vi "HFRR ADV v05.vi"() -> ()   [LabVIEW 2025] (continued)
            n2732 = Path To String(path=w3785) -> (string=w3768:string)
            n2733 = while {
              tunnel: w3777 -> [w3789]
              i -> [w3786]
              stop <- w3787 continue-if-true
              (unwired) TRUE ("line mode (F)")
              n2734 = Read from Text File "Read File"(file (use dialog)=w3789) -> (text=w3788:string)  [unwired: 3 in, 3 out]
              n2735 = local write "Numeric 16"(w3786) -> ()
              n2736 = String Length(string=w3788) -> (length=w3791:i32)
              n2737 = Greater?(x=w3791, y=1) -> (0:w3787:bool)
            }
            n2738 = local write "String 29"(w3768) -> ()
            n2739 = Search and Replace String(input string=w3768, search string=".duf", replace string=".dgf" ("replace string (\"\")")) -> (result string=→"String Indicator 4":string)  [unwired: 5 in, 3 out]
            n2740 = Match Pattern(string=w3783, regular expression=".dwm") -> (before substring=w3767:string)  [unwired: 1 in, 3 out]
            "String Indicator" <- w3767
            n2741 = Match Pattern(string=w3768, regular expression=".dwm" ("substring (\"\")")) -> (before substring=w3769:string)  [unwired: 1 in, 3 out]
            "String Indicator 3" <- w3769
            n2742 = local write "TITTLE 2"(w3767) -> ()
            n2743 = String To Path(string=w3769) -> (path=w3776:path)
            "path" <- w3776
            n2744 = call <vilib>:"Read Characters From File.vi"("file path (dialog if empty)"=w3776, "start of read offset (chars.:0)"=60 ("start of read offset (chars.: 0)")) -> ("character string"=→"String Indicator 2":string)  [unwired: 4 in, 3 out]
          }
        }
        n2745 = call <vilib>:"Query Available Printers.vi"() -> ("system configured printers"=w3468:string[])  [unwired: 9 in, 2 out]
        "System Configured Printers 2" <- w3468
        n2746 = local read "OK Button 16"() -> (w3465:bool)
        n2747 = case shown="True" "OK Button 16" {
          frame False {
          }
          frame True {
            n2748 = stacked-sequence {
              frame #0 {
                n2749 = local read "Numeric 16"() -> (w3793:i32)
                n2750 = local write "Numeric 10"(w3793) -> ()
              }
              frame #1 {
                n2751 = local read "S.NO"() -> (→"s.NO":string)
                n2752 = local read "String 29"() -> (w3797:string)
                n2753 = String To Path(string=w3797) -> (path=w3796:path)
                n2754 = Open/Create/Replace File "Open File"(file path (use dialog)=w3796) -> (refnum out=w3798:refnum<file>)  [unwired: 5 in, 2 out]
                n2755 = for {
                  N: 16 -> [_]
                  tunnel: w3798 -> [w3805]
                  i -> [w3801]
                  (unwired) TRUE ("line mode (F)")
                  n2756 = Read from Text File "Read File"(file (use dialog)=w3805) -> (text=w3799:string)  [unwired: 3 in, 3 out]
                  n2757 = Match Pattern(string=w3799, regular expression="(") -> (after substring=w3804:string)  [unwired: 1 in, 3 out]
                  n2758 = Match Pattern(string=w3804, regular expression=")") -> (before substring=w3800:string)  [unwired: 1 in, 3 out]
                  n2759 = case shown="1" w3801 {
                    tunnel: w3800 -> [w3806 w3807 _ _ w3808 w3809 w3810 w3812 w3814 w3816 w3818 w3820 w3822 w3824 _]
                    tunnel: w3799 -> [_ _ _ _ _ _ _ _ _ _ _ _ _ _ _]
                    frame 0 {
                      "TITTLE" <- w3806
                    }
                    frame 1 {
                      "Sample ID" <- w3807
                    }
                    frame 2 {
                    }
                    frame 3 {
                    }
                    frame 4 {
                      "Test Date" <- w3808
                    }
                    frame 5 {
                      "Tested by" <- w3809
                    }
                    frame 6 {
                      n2760 = Fract/Exp String To Number(string=w3810) -> (number=→"Humidity before test 2":dbl)  [unwired: 3 in, 1 out]
                    }
                    frame 7 {
                      n2761 = Fract/Exp String To Number(string=w3812) -> (number=→"Temperature before test 2":dbl)  [unwired: 3 in, 1 out]
                    }
                    frame 8 {
                      n2762 = Fract/Exp String To Number(string=w3814) -> (number=→"Humidity after test 2":dbl)  [unwired: 3 in, 1 out]
                    }
                    frame 9 {
                      n2763 = Fract/Exp String To Number(string=w3816) -> (number=→"Temperature after test 2":dbl)  [unwired: 3 in, 1 out]
                    }
                    frame 10 {
                      n2764 = Fract/Exp String To Number(string=w3818) -> (number=→"MWSD 2":dbl)  [unwired: 3 in, 1 out]
                    }
                    frame 11 {
                      n2765 = Fract/Exp String To Number(string=w3820) -> (number=→"AVP 2":dbl)  [unwired: 3 in, 1 out]
                    }
                    frame 12 {
                      n2766 = Fract/Exp String To Number(string=w3822) -> (number=→"HCF 2":dbl)  [unwired: 3 in, 1 out]
                    }
                    frame 13 {
                      n2767 = Fract/Exp String To Number(string=w3824) -> (number=→"WS1.4 2":dbl)  [unwired: 3 in, 1 out]
                    }
                    frame 14, Default {
                    }
                  }
                }
              }
              frame #2 {
              }
            }
            n2768 = local write "OK Button 16"(FALSE ("OK Button 13")) -> ()
          }
        }
        n2769 = Index Array(array=w3468, index="Select Printer 3") -> (element=w3470:string)
        "Selected Printer" <- w3470
        n2770 = case shown="True" w3465 {
          frame False {
          }
          frame True {
            n2771 = flat-sequence {
              frame #0 {
              }
              frame #1 {
                n2772 = Wait (ms)(milliseconds to wait=u32 100) -> ()  [unwired: 1 out]
              }
              frame #2 {
                n2773 = local write "OK Button 16"(FALSE ("Print 3")) -> ()
              }
            }
          }
        }
        n2774 = case shown="True" "Print" {
          tunnel: w3470 -> [_ w3762]
          frame False {
          }
          frame True {
            (unwired) i16 6 ("width (-)")
            (unwired) "TESTED BY : "
            (unwired) "TESTED DATE :"
            (unwired) "SAMPLE ID : "
            (unwired) "SAMPLE DESIGN : "
            w3720 = "\r"
            w3737 = "\r"
            # "add image"
            n2775 = local read "Sample ID"() -> (w3710:string)
            n2776 = local read "Tested by"() -> (w3713:string)
            n2777 = local read "String 34"() -> (w3700:string)
            n2778 = local read "String 45"() -> (w3680:string)
            n2779 = local read "String 35"() -> (w3695:string)
            n2780 = local read "String 37"() -> (w3693:string)
            n2781 = local read "String 32"() -> (w3715:string)
            n2782 = local read "String 36"() -> (w3690:string)
            n2783 = local read "String 31"() -> (w3714:string)
            n2784 = local read "Test Date"() -> (w3711:string)
            n2785 = local read "String 33"() -> (w3716:string)
            n2786 = local read "String 38"() -> (w3686:string)
            n2787 = local read "String 39"() -> (w3683:string)
            n2788 = local write "Print"(FALSE ("Print FF")) -> ()
            n2789 = local read "S 39"() -> (w3698:string)
            n2790 = local read "S 38"() -> (w3705:string)
            n2791 = local read "Temperature before test 2"() -> (w3736:dbl)
            n2792 = local read "Temperature after test 2"() -> (w3726:dbl)
            n2793 = local read "Humidity before test 2"() -> (w3751:dbl)
            n2794 = local read "Humidity after test 2"() -> (w3735:dbl)
            n2795 = local read "MWSD 2"() -> (w3740:dbl)
            n2796 = local read "WS1.4 2"() -> (w3718:dbl)
            n2797 = Concatenate Strings("2)" ("string"), w3700) -> (w3701:string)
            n2798 = Concatenate Strings("3)" ("string"), w3698) -> (w3699:string)
            n2799 = Concatenate Strings("1)" ("string"), w3705) -> (w3704:string)
            n2800 = Concatenate Strings("4)" ("string"), w3695) -> (w3696:string)
            n2801 = Concatenate Strings("5)" ("string"), w3693) -> (w3692:string)
            n2802 = Concatenate Strings("6)" ("string"), w3690) -> (w3689:string)
            n2803 = Concatenate Strings("7)" ("string"), w3686) -> (w3687:string)
            n2804 = Concatenate Strings("8)" ("string"), w3683) -> (w3684:string)
            n2805 = local read "HCF 2"() -> (w3722:dbl)
            n2806 = local read "AVP 2"() -> (w3739:dbl)
            n2807 = local read "s.NO"() -> (w3681:string)
            n2808 = call <vilib>:"New Report.vi"("report type"=enum16{"Standard Report", "HTML"}."Standard Report") -> ("report out"=w3760:refnum<class "NI_report.lvclass">, "error out"=w3759:errorcluster)  [unwired: 13 in]
            n2809 = local read "TITTLE"() -> (w3712:string)
            n2810 = Concatenate Strings(w3737, w3680, w3681, w3737, w3715, w3710, w3737, w3714, w3711, w3737, w3716, w3713, w3737) -> (w3730:string)
            "test by" <- w3730
            n2811 = Number To Fractional String(number=w3736, width (-)=i16 6, precision (6)=i16 2) -> (F-format string=w3725:string)  [unwired: 1 in]
            n2812 = Number To Fractional String(number=w3735, width (-)=i16 6, precision (6)=i16 2) -> (F-format string=w3738:string)  [unwired: 1 in]
            n2813 = Number To Fractional String(number=w3751, width (-)=i16 6, precision (6)=i16 2) -> (F-format string=w3756:string)  [unwired: 1 in]
            n2814 = Number To Fractional String(number=w3740, width (-)=i16 6, precision (6)=i16 2) -> (F-format string=w3742:string)  [unwired: 1 in]
            n2815 = Number To Fractional String(number=w3726, width (-)=i16 6, precision (6)=i16 2) -> (F-format string=w3727:string)  [unwired: 1 in]
            n2816 = Number To Fractional String(number=w3739, width (-)=i16 6, precision (6)=i16 2) -> (F-format string=w3741:string)  [unwired: 1 in]
            n2817 = Number To Fractional String(number=w3722, width (-)=i16 6, precision (6)=i16 2) -> (F-format string=w3721:string)  [unwired: 1 in]
            n2818 = Number To Fractional String(number=w3718, precision (6)=i16 2) -> (F-format string=w3717:string)  [unwired: 2 in]
            n2819 = call-dynamic "Set Report Header Text.vi"("report in"=w3760, "center header text"=w3712, "error in (no error)"=w3759) -> ("report out"=w3731:refnum<class "NI_report.lvclass">, "error out"=w3732:errorcluster)  [unwired: 11 in]
            n2820 = Concatenate Strings(w3720, w3704, w3756, w3720, w3701, w3725, w3720, w3699, w3738, w3720, w3696, w3727, w3720, w3692, w3742, w3720, w3689, w3741, w3720, w3687, w3721, w3720, w3684, w3717) -> (w3708:string)
            "export 2" <- w3708
            n2821 = call-poly <vilib>:"Append Report Text.vi"("report in"=w3731, "text"=w3730, "error in (no error)"=w3732) -> ("report out"=w3734:refnum<class "NI_report.lvclass">, "error out"=w3733:errorcluster)  [unwired: 9 in, 2 out]
            n2822 = local read "test by"() -> (w3707:string)
            n2823 = local read "TITTLE"() -> (w3709:string)
            n2824 = call-poly <vilib>:"Append Report Text.vi"("report in"=w3734, "error in (no error)"=w3733) -> ("report out"=w3755:refnum<class "NI_report.lvclass">, "error out"=w3753:errorcluster)  [unwired: 10 in, 2 out]
            n2825 = Concatenate Strings(w3709, w3708, w3707) -> (→"output":string)
            n2826 = call-poly <vilib>:"Append Report Text.vi"("report in"=w3755, "text"=w3708, "error in (no error)"=w3753) -> ("report out"=w3754:refnum<class "NI_report.lvclass">, "error out"=w3752:errorcluster)  [unwired: 9 in, 2 out]
            n2827 = call-dynamic "Print Report.vi"("report in"=w3754, "printer name (default)"=w3762, "error in (no error)"=w3752) -> ("report out"=w3764:refnum<class "NI_report.lvclass">, "error out"=w3765:errorcluster)  [unwired: 11 in]
            n2828 = call-dynamic "Dispose Report.vi"("report in"=w3764, "error in (no error)"=w3765) -> ()  [unwired: 13 in, 1 out]
          }
        }
        n2829 = case shown="True" "Print 2" {
          frame False {
          }
          frame True {
            n2830 = flat-sequence {
              frame #0 {
                n2831 = local read "s.NO"() -> (→"s.NO 2":string)
                n2832 = Wait (ms)(milliseconds to wait=u32 20) -> ()  [unwired: 1 out]
                n2833 = local read "Sample ID  3"() -> (→"Sample ID  6":string)
                n2834 = local read "Sample ID  4"() -> (→"Sample ID  7":string)
                n2835 = local read "Sample ID"() -> (→"Sample ID  2":string)
                n2836 = local read "Tested by"() -> (→"Tested by 2":string)
                n2837 = local read "Test Date"() -> (→"Test Date 2":string)
                n2838 = local read "Humidity after test 3"() -> (→"Humidity after test 4":dbl)
                n2839 = local read "Ref A Test Date :"() -> (→"TITTLE 4":string)
                n2840 = local read "Temperature before test 3"() -> (w3587:dbl)
                n2841 = local read "Temperature before test 3"() -> (→"Temperature after test 5":dbl)
                n2842 = local read "Temperature after test 3"() -> (→"Temperature after test 4":dbl)
                n2843 = local read "Humidity before test 3"() -> (→"Humidity before test 4":dbl)
                n2844 = local write "Temperature before test 3"(w3587) -> ()
                n2845 = local read "image data"() -> (w3578:T11)
                n2846 = String To Path(string="C:\\LAB-IQ\\im\\Temp_resized.jpg") -> (path=w3579:path)
                "path 2" <- w3579
                n2847 = call <vilib>:"Write JPEG File.vi"("image data"=w3578, "path to JPEG file"=w3579) -> ()  [unwired: 8 in, 2 out]
                "Ref A Test Date :" <- "Ref A Test Date :"
                "Ref B Test Date :" <- "Ref B Test Date :"
                "Ref B Scar Value :" <- "Ref B Scar Value :"
                "Ref A Scar Value :" <- "Ref A Scar Value :"
              }
              frame #1 {
                (unwired) HTML_Report_Image_Alignment."MIDDLE" ("alignment (default)")
                w3615 = u16 0 items=["portrait", "landscape"] ("orientation (portrait)")
                (unwired) HTML_Report_Image_Alignment."ABSMIDDLE" ("alignment (default)")
                (unwired) "TESTED BY : "
                (unwired) "TESTED DATE :"
                (unwired) "SAMPLE ID : "
                (unwired) "SAMPLE DESIGN : "
                w3648 = "\r"
                # "add image"
                n2848 = Wait (ms)(milliseconds to wait=u32 20) -> ()  [unwired: 1 out]
                n2849 = local read "Sample ID  2"() -> (w3641:string)
                n2850 = local read "Wear Scar X"() -> (w3613:dbl)
                "Length ( microns ) 2" <- w3613
                n2851 = local read "Wear Scar Y"() -> (w3612:dbl)
                "Wear Scar Y ( microns ) :" <- w3612
                n2852 = local read "Test Date 2"() -> (w3642:string)
                n2853 = local read "Tested by 2"() -> (w3643:string)
                n2854 = local read "String 46"() -> (w3639:string)
                n2855 = local read "String 48"() -> (w3645:string)
                n2856 = local read "String 47"() -> (w3644:string)
                n2857 = local read "String 49"() -> (w3646:string)
                n2858 = local read "String 10"() -> (w3599:string)
                n2859 = local read "s.NO 2"() -> (w3640:string)
                n2860 = Add(x=w3613, y=w3612) -> (x+y=w3611:dbl)
                n2861 = call <vilib>:"New Report.vi"("report type"=enum16{"Standard Report", "HTML"}."HTML") -> ("report out"=w3619:refnum<class "NI_report.lvclass">, "error out"=w3617:errorcluster)  [unwired: 13 in]
                n2862 = Concatenate Strings(w3648, w3639, w3640, w3648, w3645, w3641, w3648, w3644, w3642, w3648, w3646, w3643, w3648) -> (→"test by 2":string)
                n2863 = Concatenate Strings("C:\\LAB-IQ\\Data\\" ("string"), w3599, ".jpg" ("string")) -> ()  [unwired: 1 out]
                n2864 = Divide(x=w3611, y=2.0) -> (x/y=→"Mean Wear ( microns) :":dbl)
                n2865 = call-dynamic "Set Report Orientation.vi"("report in"=w3619, "orientation (portrait)"=w3615, "error in (no error)"=w3617) -> ("report out"=w3618:refnum<class "NI_report.lvclass">, "error out"=w3616:errorcluster)  [unwired: 11 in]
                n2866 = for {
                  N: 5 -> [_]
                  tunnel: w3618 -> [w3669]
                  tunnel: [w3668] -> w3597
                  tunnel: w3616 -> [w3667]
                  tunnel: [w3666] -> w3596
                  n2867 = call-dynamic "Set Report Tab Width.vi"("report in"=w3669, "error in (no error)"=w3667) -> ("report out"=w3668:refnum<class "NI_report.lvclass">, "error out"=w3666:errorcluster)  [unwired: 12 in]
                }
                n2868 = local read "TITTLE"() -> (w3614:string)
                n2869 = call-dynamic "Set Report Header Text.vi"("report in"=w3597, "center header text"=w3614, "error in (no error)"=w3596) -> ("report out"=w3635:refnum<class "NI_report.lvclass">, "error out"=w3634:errorcluster)  [unwired: 11 in]
                n2870 = for {
                  N: 1 -> [_]
                  tunnel: [w3673] -> w3621
                  tunnel: [w3672] -> w3620
                  tunnel: w3635 -> [w3671]
                  tunnel: w3634 -> [w3670]
                  n2871 = call-dynamic "New Report Line.vi"("report in"=w3671, "error in (no error)"=w3670) -> ("report out"=w3673:refnum<class "NI_report.lvclass">, "error out"=w3672:errorcluster)  [unwired: 12 in]
                }
                n2872 = for {
                  N: 2 -> [_]
                  tunnel: [w3665] -> w3627
                  tunnel: [w3664] -> w3626
                  tunnel: w3621 -> [w3663]
                  tunnel: w3620 -> [w3662]
                  n2873 = call-dynamic "New Report Line.vi"("report in"=w3663, "error in (no error)"=w3662) -> ("report out"=w3665:refnum<class "NI_report.lvclass">, "error out"=w3664:errorcluster)  [unwired: 12 in]
                }
                n2874 = for {
                  N: 25 -> [_]
                  tunnel: w3627 -> [w3661]
                  tunnel: w3626 -> [w3659]
                  tunnel: [w3660] -> w3630
                  tunnel: [w3658] -> w3629
                  n2875 = call-dynamic "Set Report Tab Width.vi"("report in"=w3661, "error in (no error)"=w3659) -> ("report out"=w3660:refnum<class "NI_report.lvclass">, "error out"=w3658:errorcluster)  [unwired: 12 in]
                }
                n2876 = control-ref of="Tab Control 9"() -> (w3625:refnum<vi>)
                n2877 = call-dynamic "Append Control Image to Report.vi"("report in"=w3630, "alignment (default)"=HTML_Report_Image_Alignment."ABSMIDDLE", "ctrl reference"=w3625, "error in (no error)"=w3629) -> ("report out"=w3624:refnum<class "NI_report.lvclass">, "error out"=w3623:errorcluster)  [unwired: 8 in, 2 out]
                n2878 = for {
                  N: 3 -> [_]
                  tunnel: [w3657] -> w3608
                  tunnel: [w3656] -> w3607
                  tunnel: w3624 -> [w3655]
                  tunnel: w3623 -> [w3654]
                  n2879 = call-dynamic "New Report Line.vi"("report in"=w3655, "error in (no error)"=w3654) -> ("report out"=w3657:refnum<class "NI_report.lvclass">, "error out"=w3656:errorcluster)  [unwired: 12 in]
                }
                n2880 = for {
                  N: 100 -> [_]
                  tunnel: w3608 -> [w3653]
                  tunnel: w3607 -> [w3651]
                  tunnel: [w3652] -> w3604
                  tunnel: [w3650] -> w3602
                  n2881 = call-dynamic "Set Report Tab Width.vi"("report in"=w3653, "error in (no error)"=w3651) -> ("report out"=w3652:refnum<class "NI_report.lvclass">, "error out"=w3650:errorcluster)  [unwired: 12 in]
                }
                n2882 = String To Path(string="C:\\LAB-IQ\\im\\Temp_resized.jpg") -> (path=w3594:path)
                n2883 = call-poly <vilib>:"Append Image to Report.vi"("report in"=w3604, "path or URL of image"=w3594, "error in (no error)"=w3602) -> ("report out"=w3603:refnum<class "NI_report.lvclass">, "error out"=w3601:errorcluster)  [unwired: 9 in, 2 out]
                n2884 = call-poly <vilib>:"Open HTML Report in Browser.vi"("report in"=w3603, "error in (no error)"=w3601) -> ("report out"=w3638:refnum<class "NI_report.lvclass">, "error out"=w3637:errorcluster)  [unwired: 11 in, 1 out]
                n2885 = call-dynamic "Dispose Report.vi"("report in"=w3638, "error in (no error)"=w3637) -> ()  [unwired: 13 in, 1 out]
              }
              frame #2 {
              }
              frame #3 {
                n2886 = disable-structure shown="Disabled" {
                  frame Disabled {
                    n2887 = local read "String 10"() -> (w3678:string)
                    n2888 = Concatenate Strings("C:\\LAB-IQ-NXT\\Data\\" ("string"), w3678, ".jpg" ("string")) -> (w3676:string)
                    n2889 = String To Path(string=w3676) -> (path=w3675:path)
                    n2890 = Delete(path (use dialog)=w3675) -> ()  [unwired: 4 in, 3 out]
                  }
                  frame Enabled {
                  }
                }
                n2891 = local write "Print 2"(FALSE ("Print")) -> ()
              }
            }
          }
        }
      }
    }
    n2892 = property on="SetTemp" class="DigNum (strict)"("Disabled"=w1629) -> ()  [unwired: 2 in, 2 out]
    n2893 = Multiply(x=w1619, y=w1621) -> (x*y=w1620:dbl)
    n2894 = local read "MWSD"() -> (w1618:dbl)
    n2895 = Add(x=w1620, y=w1618) -> (x+y=→"WS1.4":dbl)
    n2896 = Wait (ms)(milliseconds to wait=u32 50) -> ()  [unwired: 1 out]
    n2897 = Wait (ms)(milliseconds to wait=u32 50) -> ()  [unwired: 1 out]
    n2898 = local read "Quit"() -> (w1617:bool)
  }
  n2899 = VISA Close(VISA resource name=w52, error in (no error)=w51) -> (error out=w49:errorcluster)
  n2900 = call <vilib>:"Clear Errors.vi"("error in (no error)"=w49) -> ()  [unwired: 5 in, 2 out]
  n2901 = VISA Close(VISA resource name=w37, error in (no error)=w36) -> ()  [unwired: 1 out]
  n2902 = while {
    tunnel: [w3837] -> w46
    shift-right: [w3830] -> _
    shift-left: 0.0 -> [w3833]
    shift-right: [w3829] -> _
    shift-left: 0.0 -> [w3832]
    shift-right: [w3828] -> _
    shift-left: 400.0 ("vc_cmd") -> [w3831]
    stop <- w3837 stop-if-true
    # "PID LOGIC"
    n2903 = local read "RUN"() -> (w3835:bool)
    n2904 = local read "Auto Start Test"() -> (w3834:bool)
    n2905 = local read "START TEMP"() -> (w3826:bool)
    n2906 = Or(x=w3835, y=w3834) -> (x .or. y?=w3836:bool)
    n2907 = And(x=w3836, y=w3826) -> (x .and. y?=w3827:bool)
    n2908 = Wait (ms)(milliseconds to wait=u32 20) -> ()  [unwired: 1 out]
    n2909 = case shown="True" w3827 {
      tunnel: [400.0 ("out_vc_cmd") w3857] -> w3828
      tunnel: [w3840 w3859] -> w3829
      tunnel: [w3840 w3858] -> w3830
      tunnel: w3833 -> [_ w3847]
      tunnel: w3832 -> [_ w3846]
      tunnel: w3831 -> [_ w3845]
      frame False {
        w3840 = 0.0 ("error_out")
      }
      frame True {
        n2910 = local read "measured_stroke"() -> (w3848:dbl)
        n2911 = local read "Set Strk"() -> (w3842:dbl)
        n2912 = Add(x=w3842, y="STROKE ADD") -> (x+y=w3843:dbl)
        n2913 = formula code="// Zero-Hardcode Explicit Positional-Form PID Engine\n// Inputs: target_stroke, measured_stroke, dt, prev_error, integral_accumulator_in, prev_vc_cmd\n//         kp, ki, kd, max_step_change, max_amplitude, min_amplitude, startup_cmd\n// Outputs: vc_cmd, error_out, out_error, integral_accumulator_out, out_vc_cmd\n\n// 1. Calculate Tracking Error\nfloat current_error = target_stroke - measured_stroke;\nerror_out = current_error;\n\n// 2. Compute Proportional Term\nfloat p_term = kp * current_error;\n\n// 3. Compute Derivative Term\nfloat d_term = 0.0;\nif (dt > 0.0) {\n    d_term = kd * ((current_error - prev_error) / dt);\n}\n\n// 4. Update and Accumulate Integral Term\nfloat current_integral = integral_accumulator_in + (current_error * dt);\nfloat i_term = ki * current_integral;\n\n// 5. Calculate Ideal Target Command\nfloat ideal_command = startup_cmd + p_term + i_term + d_term;\n\n// 6. Anti-Windup Protection (Back-calculation method)\nif (ideal_command > max_amplitude) {\n    float excess = ideal_command - max_amplitude;\n    if (ki > 0.0) {\n        current_integral -= excess / ki;\n    }\n    ideal_command = max_amplitude;\n} else if (ideal_command < min_amplitude) {\n    float excess = ideal_command - min_amplitude;\n    if (ki > 0.0) {\n        current_integral -= excess / ki;\n    }\n    ideal_command = min_amplitude;\n}\n\n// 7. Apply Loop Rate Limiting (Protects voice coil from large voltage steps)\nfloat raw_adjustment = ideal_command - prev_vc_cmd;\n\nif (raw_adjustment > max_step_change) {\n    raw_adjustment = max_step_change;\n} else if (raw_adjustment < -max_step_change) {\n    raw_adjustment = -max_step_change;\n}\n\nfloat next_vc_cmd = prev_vc_cmd + raw_adjustment;\n\n// Final Output Safety Safeguard Clamping\nif (next_vc_cmd > max_amplitude) {\n    next_vc_cmd = max_amplitude;\n} else if (next_vc_cmd < min_amplitude) {\n    next_vc_cmd = min_amplitude;\n}\n\n// 8. Map to Shift Registers for memory persistence\nvc_cmd = next_vc_cmd;\nout_error = current_error;                     \nintegral_accumulator_out = current_integral;  \nout_vc_cmd = next_vc_cmd;"("target_stroke"=w3843, "measured_stroke"=w3848, "dt"="dt", "integral_accumulator_in"=w3846, "prev_error"=w3847, "prev_vc_cmd"=w3845, "kp"="kp", "ki"="ki", "kd"="kd", "max_step_change"="max_step_change", "max_amplitude"="max_amplitude", "min_amplitude"="min_amplitude", "startup_cmd"="startup_cmd") -> ("vc_cmd"=w3863:dbl, "out_error"=w3858:dbl, "integral_accumulator_out"=w3859:dbl, "out_vc_cmd"=w3857:dbl)  [unwired: 1 out]
        "output Vpp" <- w3863
        n2914 = Number To Fractional String(number=w3863, precision (6)=i16 1) -> (F-format string=w3861:string)  [unwired: 2 in]
        n2915 = Concatenate Strings("DAC;" ("string"), w3861) -> (w3844:string)
        n2916 = local write "Command"(w3844) -> ()
        "prev_error" <- w3847
        "integral_accumulator_in" <- w3846
        "prev_vc_cmd" <- w3845
      }
    }
    n2917 = local read "Quit"() -> (w3837:bool)
  }
  n2918 = Or(x=w42, y=w41) -> (x .or. y?=w43:bool)
  n2919 = Or(x=w39, y=w43) -> (x .or. y?=w48:bool)
  n2920 = control-ref of="new picture"() -> ()  [unwired: 1 out]
  n2921 = Or(x=w54, y=w48) -> (x .or. y?=w45:bool)
  n2922 = Or(x=w45, y=w46) -> (x .or. y?=w40:bool)
  n2923 = while {
    tunnel: [w3864] -> w53
    i -> [w3871]
    stop <- w3864 stop-if-true
    n2924 = local read "Quit"() -> (w3864:bool)
    n2925 = Equal To 0?(x=w3871) -> (x = 0?=w3869:bool)
    n2926 = call "Elapsed Time3"("Time Target (s)"=45.0, "Auto Reset"=TRUE) -> ("Time has Elapsed"=w3868:bool)  [unwired: 10 in, 7 out]
    n2927 = Wait (ms)(milliseconds to wait=u32 50) -> ()  [unwired: 1 out]
    n2928 = Or(x=w3868, y=w3869) -> (x .or. y?=w3870:bool)
    n2929 = case shown="True" w3870 {
      frame False {
      }
      frame True {
        n2930 = call <vilib>:"System Exec.vi"("run minimized? (F)"=TRUE, "error in (no error)"="error in (no error)", "command line"="powercfg.exe -change -monitor-timeout-ac 0") -> ("error out"=w3882:errorcluster)  [unwired: 5 in, 3 out]
        n2931 = call <vilib>:"System Exec.vi"("run minimized? (F)"=TRUE, "error in (no error)"=w3882, "command line"="powercfg.exe -change -disk-timeout-ac 0") -> ("error out"=w3881:errorcluster)  [unwired: 5 in, 3 out]
        n2932 = call <vilib>:"System Exec.vi"("run minimized? (F)"=TRUE, "error in (no error)"=w3881, "command line"="powercfg.exe -change -standby-timeout-ac 0") -> ("error out"=w3880:errorcluster)  [unwired: 5 in, 3 out]
        n2933 = call <vilib>:"System Exec.vi"("run minimized? (F)"=TRUE, "error in (no error)"=w3880, "command line"="powercfg.exe -change -hibernate-timeout-ac 0") -> ("error out"=w3879:errorcluster)  [unwired: 5 in, 3 out]
        n2934 = call <vilib>:"Simple Error Handler.vi"("error in (no error)"=w3879) -> ("error out"=w3885:errorcluster)  [unwired: 4 in, 4 out]
        n2935 = call <vilib>:"Clear Errors.vi"("error in (no error)"=w3885) -> ("error out"=→"error out":errorcluster)  [unwired: 5 in, 1 out]
      }
    }
  }
  n2936 = Compound Arithmetic op=OR(w56, w40, w53) -> (w55:bool)
  n2937 = flat-sequence {
    tunnel: w55 -> [_]
    tunnel: [w3887] -> w17
    tunnel: w17 -> [_]
    frame #0 {
      n2938 = call "CLOSE CONNECTION.vi"() -> ("error out"=w3887:errorcluster)  [unwired: 11 in]
    }
    frame #1 {
      n2939 = Quit LabVIEW(quit? (T)=TRUE) -> ()
      n2940 = local write "Quit"(FALSE ("EXIT")) -> ()
    }
  }
  n2941 = property on="Heater Button" class="Bool (strict)"("Visible"=TRUE) -> ()  [unwired: 2 in, 2 out]
  n2942 = disable-structure shown="Disabled" {
    disable-tunnel: _ -> [w3893 _]
    disable-tunnel: _ -> [w3890 _]
    disable-tunnel: _ -> [w3891 _]
    frame Disabled {
      n2943 = disable-structure shown="Disabled" {
        disable-tunnel: [w3900 _] -> w3892
        frame Disabled {
          n2944 = while {
            shift-right: [w3942] -> w3898
            shift-left: errorcluster {"status"=TRUE, "code"=0, "source"="Init"} ("error out") -> [w3907]
            shift-right: [w3941] -> w3897
            shift-left: _ -> [w3908]
            shift-right: [w3940] -> _
            shift-left: "" -> [w3939]
            tunnel: [w3901] -> w3900
            shift-right: ["Set Rh"] -> _
            shift-left: 0.0 ("Set Rh") -> [w3933]
            tunnel: [w3910] -> _
            i -> [w3910]
            stop <- w3901 stop-if-true
            n2945 = flat-sequence {
              tunnel: w3907 -> [w3945]
              tunnel: [w3945] -> w3906
              frame #0 {
                n2946 = Wait (ms)(milliseconds to wait=u32 200) -> ()  [unwired: 1 out]
              }
            }
            n2947 = local read "Com Port 3"() -> (w3909:refnum<visa-resource-name>)
            n2948 = local read "Humidity Str Rec"() -> (w3911:string)
            n2949 = Not Equal?(x="Set Rh", y=w3933) -> (x != y?=w3938:bool)
            n2950 = Number To Decimal String(number="Set Rh") -> (decimal integer string=w3936:string)  [unwired: 1 in]
            n2951 = Not Equal?(x=w3909, y=w3908) -> (x != y?=w3904:bool)
            n2952 = Concatenate Strings("#setPoint00" ("string"), w3936) -> (w3937:string)
            n2953 = case shown="False" w3938 {
              tunnel: w3937 -> [_ w3957]
              frame False {
                n2954 = local read "Humidity"() -> (w3954:bool)
                n2955 = case shown="True" w3954 {
                  frame False {
                    n2956 = local write "Humidity Str Send"("stop" ("Humidity Str Send")) -> ()
                  }
                  frame True {
                    n2957 = local write "Humidity Str Send"("start" ("Humidity Str Send")) -> ()
                  }
                }
              }
              frame True {
                n2958 = local write "Humidity Str Send"(w3957) -> ()
              }
            }
            n2959 = Or(x=w3904) -> (y=w3902:bool, x .or. y?=w3903:bool)
            n2960 = String Subset(string=w3911, offset (0)=7) -> (substring=w3926:string)  [unwired: 1 in]
            n2961 = Match Pattern(string=w3911, regular expression="?") -> (offset past match=w3929:i32)  [unwired: 1 in, 3 out]
            n2962 = Match Pattern(string=w3911, regular expression="v") -> (offset past match=w3932:i32)  [unwired: 1 in, 3 out]
            n2963 = case shown="True" w3903 {
              tunnel: w3906 -> [w3943 _]
              tunnel: [w3943 errorcluster {"status"=TRUE, "code"=0, "source"="Init"} ("error out")] -> w3905
              frame False {
              }
              frame True {
              }
            }
            n2964 = Equal?(x=w3929, y=-1) -> (x = y?=w3913:bool)
            n2965 = Match Pattern(string=w3926, regular expression="g") -> (after substring=w3927:string, offset past match=w3918:i32)  [unwired: 1 in, 2 out]
            n2966 = Match Pattern(string=w3926, regular expression="y") -> (after substring=w3925:string, offset past match=w3919:i32)  [unwired: 1 in, 2 out]
            n2967 = Greater?(x=w3919, y=w3918) -> (0:w3924:bool)
            n2968 = Greater Or Equal To 0?(x=w3919) -> (x >= 0?=w3916:bool)
            n2969 = Greater Or Equal To 0?(x=w3918) -> (x >= 0?=w3917:bool)
            n2970 = Or(x=w3916, y=w3917) -> (x .or. y?=w3915:bool)
            n2971 = Greater Or Equal To 0?(x=w3932) -> (x >= 0?=w3914:bool)
            n2972 = Select(t=w3925, s=w3924, f=w3927) -> (s? t:f=w3920:string)
            n2973 = case shown="Error" w3905 {
              selector: w3905 -> [w3970 w4016]
              tunnel: [w3968 w4009] -> w3942
              tunnel: w3908 -> [w3971 w4015]
              tunnel: [w3969 w4018] -> w3941
              tunnel: w3939 -> [w3958 w4017]
              tunnel: [w3965 w4017] -> w3940
              frame No Error {
                n2974 = call "Elapsed Time7"() -> ("Time has Elapsed"=w3964:bool)  [unwired: 12 in, 7 out]
                n2975 = Not Equal?(x="Humidity Str Send", y=w3958) -> (x != y?=w3960:bool)
                n2976 = Or(x=w3960, y=w3964) -> (x .or. y?=w3963:bool)
                n2977 = Select(t="Humidity Str Send", s=w3960, f="vals" ("regular expression")) -> (s? t:f=w3959:string)
                n2978 = Or(x=w3963, y="Send") -> (x .or. y?=w3967:bool)
                n2979 = case shown="True" w3967 {
                  tunnel: [w3974 w3979] -> w3968
                  tunnel: w3971 -> [w3973 w3987]
                  tunnel: w3970 -> [w3974 w3986]
                  tunnel: [w3973 w3980] -> w3969
                  tunnel: w3959 -> [_ w3985]
                  tunnel: [w3972 w3976] -> w3965
                  tunnel: "Humidity Str Send" -> [_ w3977]
                  tunnel: w3960 -> [_ w3978]
                  tunnel: w3958 -> [w3972 w3975]
                  frame False {
                  }
                  frame True {
                    n2980 = flat-sequence {
                      tunnel: w3987 -> [w3995]
                      tunnel: w3986 -> [w3994]
                      tunnel: w3985 -> [w3991]
                      tunnel: [w3993] -> w3984
                      tunnel: [w3992] -> w3983
                      tunnel: w3984 -> [w3998]
                      tunnel: w3983 -> [w3997]
                      tunnel: [w3998] -> w3982
                      tunnel: [w3997] -> w3981
                      tunnel: w3982 -> [w4005]
                      tunnel: w3981 -> [w4004]
                      tunnel: [w4003] -> w3980
                      tunnel: [w4002] -> w3979
                      frame #0 {
                        n2981 = local write "Ser Led"(TRUE ("Boolean 4")) -> ()
                        n2982 = Concatenate Strings(w3991, "\r") -> (w3990:string)
                        n2983 = VISA Write(VISA resource name=w3995, write buffer=w3990, error in (no error)=w3994) -> (VISA resource name out=w3993:refnum<visa-resource-name>, error out=w3992:errorcluster)  [unwired: 1 out]
                      }
                      frame #1 {
                        n2984 = Wait (ms)(milliseconds to wait="wait") -> ()  [unwired: 1 out]
                      }
                      frame #2 {
                        w4000 = FALSE ("Send")
                        n2985 = property class="Instr"(reference=w4005, error in=w4004) -> (reference out=w4006:refnum<visa-resource-name>, error out=w4007:errorcluster, "Serial Settings:Number of Bytes at Serial Port"=w3999:u32)
                        n2986 = local write "Send"(w4000) -> ()
                        n2987 = local write "Ser Led"(w4000) -> ()
                        n2988 = VISA Read(VISA resource name=w4006, byte count=w3999, error in (no error)=w4007) -> (VISA resource name out=w4003:refnum<visa-resource-name>, read buffer=→"Humidity Str Rec":string, error out=w4002:errorcluster)  [unwired: 1 out]
                      }
                    }
                    n2989 = Select(t=w3977, s=w3978, f=w3975) -> (s? t:f=w3976:string)
                  }
                }
              }
              frame Error {
                w4023 = u16 0 items=["None"=0, "XON/XOFF"=1, "RTS/CTS"=2, "DTR/DSR"=4] ("flow control")
                w4019 = u16 0 items=["None", "Odd", "Even", "Mark", "Space"] ("parity")
                w4022 = u16 10 items=["1.0"=10, "1.5"=15, "2.0"=20] ("stop bits")
                n2990 = VISA Close(VISA resource name=w4015, error in (no error)=w4016) -> (error out=w4014:errorcluster)
                n2991 = local write "humid"("" ("humid")) -> ()
                n2992 = local write "Humidity Str Rec"("" ("Humidity Str Rec")) -> ()
                n2993 = call <vilib>:"Clear Errors.vi"("error in (no error)"=w4014) -> ("error out"=w4013:errorcluster)  [unwired: 5 in, 1 out]
                n2994 = local read "Com Port 3"() -> (w4012:refnum<visa-resource-name>)
                n2995 = call-poly "VISA Configure Serial Port"("VISA resource name"=w4012, "timeout (10sec)"=u32 1000, "termination char\n(0xA = '\\n' = LF)"=u8 10 ("termination char\n(0xA = '\\n' = LF)"), "Enable Termination\nChar (T)"=FALSE ("Enable Termination Char (T)"), "data bits (8)"=u16 8 ("data bits"), "parity (0:none)"=w4019, "error in (no error)"=w4013, "stop bits (10: 1 bit)"=w4022, "flow control (0:none)"=w4023) -> ("VISA resource name out"=w4018:refnum<visa-resource-name>, "baud rate (9600)"=w4010:u32, "error out"=w4009:errorcluster)  [unwired: 4 in]
              }
            }
            n2996 = Compound Arithmetic op=AND(w3914, w3913, w3915) -> (w3912:bool)
            n2997 = case shown="True" w3912 {
              tunnel: w3911 -> [_ _]
              tunnel: w3920 -> [_ w3950]
              frame False {
              }
              frame True {
                w3948 = " " ("regular expression")
                n2998 = Match Pattern(string=w3950, regular expression=" ") -> (after substring=w3952:string)  [unwired: 1 in, 3 out]
                n2999 = Match Pattern(string=w3952, regular expression=w3948) -> (before substring=→"humid":string, after substring=w3949:string)  [unwired: 1 in, 2 out]
                n3000 = Match Pattern(string=w3949, regular expression=w3948) -> (before substring=→"temp_@Rh sensor":string)  [unwired: 1 in, 3 out]
              }
            }
            n3001 = local read "Quit"() -> (w3901:bool)
          }
          n3002 = VISA Close(VISA resource name=w3897, error in (no error)=w3898) -> (error out=w3894:errorcluster)
          n3003 = call <vilib>:"Clear Errors.vi"("error in (no error)"=w3894) -> ()  [unwired: 5 in, 2 out]
        }
        frame Enabled {
        }
      }
    }
    frame Enabled {
    }
  }
  n3004 = while {
    tunnel: [w4030] -> _
    i -> [w4030]
    stop <- w4026 stop-if-true
    # "Langauage selection"
    n3005 = Equal?(x="Lan flag", y=22.0) -> ()  [unwired: 1 out]
    n3006 = disable-structure shown="Disabled" {
      frame Disabled {
        n3007 = stacked-sequence {
          frame #0 {
            n3008 = case shown="\"Russian\"" "Language Selection" {
              tunnel: [0 1] -> w4032
              frame "English", Default {
              }
              frame "Russian" {
              }
            }
            n3009 = for {
              N: 130 -> [_]
              tunnel: "Table" -> [w4041]
              tunnel: w4032 -> [w4040]
              i -> [w4039]
              n3010 = Index Array(array=w4041, index (row)=w4039, index (col)=w4040) -> (element=w4038:string)
              n3011 = case shown="123" w4039 {
                tunnel: w4038 -> [w4042 w4043 _ w4044 w4045 w4046 w4047 w4048 w4049 w4050 w4051 w4052 w4053 w4054 w4055 w4056 w4057 w4058 w4059 w4060 w4061 w4062 w4063 w4064 w4065 w4066 w4067 w4068 w4069 _ _ w4070 w4071 w4072 w4073 w4074 w4075 w4084 w4091 w4098 w4105 w4109 w4112 w4115 w4117 w4119 w4120 w4121 w4122 w4123 w4124 w4125 w4126 w4127 w4128 w4129 w4130 w4131 w4132 w4133 w4134 w4135 w4136 w4137 w4138 w4139 w4140 w4141 w4142 w4143 w4144 w4145 w4146 w4147 w4148 w4149 w4150 w4151 w4152 w4153 w4154 w4155 w4156 w4157 w4158 w4159 w4160 w4161 w4162 w4163 w4164 w4165 w4166 w4167 w4168 w4169 w4170 w4171 w4172 w4173 w4174 w4175 w4176 w4177 w4178 _ w4179 w4180 w4181 w4182 w4183 w4184 w4185 w4186 w4187 w4188 w4189 w4190 w4191 _ w4192 w4193 w4194 w4195 w4196 w4197 _]
                frame 0 {
                  n3012 = local write "S"(w4042) -> ()
                }
                frame 1 {
                  n3013 = local write "S 2"(w4043) -> ()
                }
                frame 2 {
                }
                frame 3 {
                  n3014 = local write "S 4"(w4044) -> ()
                }
                frame 4 {
                  n3015 = property on="FILE" class="Str"("Caption.Text"=w4045) -> ()  [unwired: 2 in, 2 out]
                }
                frame 5 {
                  n3016 = property on="Fuel Discription :" class="Str"("Caption.Text"=w4046) -> ()  [unwired: 2 in, 2 out]
                }
                frame 6 {
                  n3017 = property on="Remarks :" class="Str"("Caption.Text"=w4047) -> ()  [unwired: 2 in, 2 out]
                }
                frame 7 {
                  n3018 = property on="Save & Continue" class="Bool (strict)"("Boolean Text.Text"=w4048) -> ()  [unwired: 2 in, 2 out]
                }
                frame 8 {
                }
                frame 9 {
                  n3019 = property on="Set Hz" class="DigNum (strict)"("Caption.Text"=w4050) -> ()  [unwired: 2 in, 2 out]
                }
                frame 10 {
                  "String 3" <- w4051
                }
                frame 11 {
                  n3020 = property on="NORMAL LOAD" class="DigNum (strict)"("Caption.Text"=w4052) -> ()  [unwired: 2 in, 2 out]
                }
                frame 12 {
                  "String 5" <- w4053
                }
                frame 13 {
                  n3021 = property on="Set Temp" class="DigNum (strict)"("Caption.Text"=w4054) -> ()  [unwired: 2 in, 2 out]
                }
                frame 14 {
                  n3022 = local write "S 15"(w4055) -> ()
                }
                frame 15 {
                  n3023 = property on="Set Rh" class="DigNum (strict)"("Caption.Text"=w4056) -> ()  [unwired: 2 in, 2 out]
                }
                frame 16 {
                  "String 13" <- w4057
                  "String 26" <- w4057
                }
                frame 17 {
                  n3024 = local write "S 18"(w4058) -> ()
                }
                frame 18 {
                  "String 17" <- w4059
                }
                frame 19 {
                  n3025 = property on="test time" class="DigNum (strict)"("Caption.Text"=w4060) -> ()  [unwired: 2 in, 2 out]
                }
                frame 20 {
                  "String 18" <- w4061
                  "String 22" <- w4061
                }
                frame 21 {
                  n3026 = property on="Elapsed time" class="DigNum (strict)"("Caption.Text"=w4062) -> ()  [unwired: 2 in, 2 out]
                }
                frame 22 {
                  n3027 = property on="Samplingtime 2" class="DigNum (strict)"("Caption.Text"=w4063) -> ()  [unwired: 2 in, 2 out]
                }
                frame 23 {
                  "String 21" <- w4064
                }
                frame 24 {
                  n3028 = property on="Countdown" class="DigNum (strict)"("Caption.Text"=w4065) -> ()  [unwired: 2 in, 2 out]
                }
                frame 25 {
                  n3029 = property on="Countdown 2" class="DigNum (strict)"("Caption.Text"=w4066) -> ()  [unwired: 2 in, 2 out]
                }
                frame 26 {
                  n3030 = property on="Engage" class="Bool (strict)"("Boolean Text.Text"=w4067) -> ()  [unwired: 2 in, 2 out]
                }
                frame 27 {
                  n3031 = property on="Boolean  4" class="Bool (strict)"("Boolean Text.Text"=w4068) -> ()  [unwired: 2 in, 2 out]
                }
                frame 28 {
                  n3032 = property on="Test \nStatus" class="Bool (strict)"("Boolean Text.Text"=w4069) -> ()  [unwired: 2 in, 2 out]
                }
                frame 29 {
                }
                frame 30 {
                }
                frame 31 {
                }
                frame 32 {
                  n3033 = property on="RSTCOF" class="Bool"("Boolean Text.Text"=w4071) -> ()  [unwired: 2 in, 2 out]
                  n3034 = property on="RST FF" class="Bool"("Boolean Text.Text"=w4071) -> ()  [unwired: 2 in, 2 out]
                  n3035 = property on="RST TEMP" class="Bool"("Boolean Text.Text"=w4071) -> ()  [unwired: 2 in, 2 out]
                  n3036 = property on="RSTV1 3" class="Bool"("Boolean Text.Text"=w4071) -> ()  [unwired: 2 in, 2 out]
                  n3037 = property on="rstv2" class="Bool"("Boolean Text.Text"=w4071) -> ()  [unwired: 2 in, 2 out]
                  n3038 = property on="RSTV1 2" class="Bool"("Boolean Text.Text"=w4071) -> ()  [unwired: 2 in, 2 out]
                  n3039 = property on="RST CP" class="Bool"("Boolean Text.Text"=w4071) -> ()  [unwired: 2 in, 2 out]
                }
                frame 33 {
                  "S 61" <- w4072
                }
                frame 34 {
                  "String 23" <- w4073
                }
                frame 35 {
                  n3040 = property on="Rh Before" class="DigNum (strict)"("Caption.Text"=w4074) -> ()  [unwired: 2 in, 2 out]
                }
                frame 36 {
                  n3041 = Match Pattern(string=w4075, regular expression=",") -> (before substring=→"bs":string, after substring=→"as":string)  [unwired: 1 in, 2 out]
                  n3042 = property on="Rh After" class="DigNum (strict)"("Caption.Text"=w4075) -> ()  [unwired: 2 in, 2 out]
                }
                frame 37 {
                  n3043 = Match Pattern(string=w4084, regular expression=",") -> (before substring=w4083:string, after substring=w4082:string)  [unwired: 1 in, 2 out]
                  "bs" <- w4083
                  "as" <- w4082
                  n3044 = Concatenate Strings(w4083, w4082) -> (w4079:string)
                  n3045 = property on="Humidity before test 2" class="DigNum (strict)"("Caption.Text"=w4079) -> ()  [unwired: 2 in, 2 out]
                  n3046 = property on="Humidity before test" class="DigNum (strict)"("Caption.Text"=w4079) -> ()  [unwired: 2 in, 2 out]
                  n3047 = Concatenate Strings(w4079, "=" ("string")) -> (w4080:string)
                  n3048 = local write "S 38"(w4080) -> ()
                }
                frame 38 {
                  n3049 = Match Pattern(string=w4091, regular expression=",") -> (before substring=w4090:string, after substring=w4089:string)  [unwired: 1 in, 2 out]
                  "bs" <- w4090
                  "as" <- w4089
                  n3050 = Concatenate Strings(w4090, w4089) -> (w4086:string)
                  n3051 = property on="Humidity after test 2" class="DigNum (strict)"("Caption.Text"=w4086) -> ()  [unwired: 2 in, 2 out]
                  n3052 = Concatenate Strings(w4086, "=" ("string")) -> (w4088:string)
                  n3053 = property on="Humidity after test" class="DigNum (strict)"("Caption.Text"=w4086) -> ()  [unwired: 2 in, 2 out]
                  n3054 = local write "S 39"(w4088) -> ()
                }
                frame 39 {
                  n3055 = Match Pattern(string=w4098, regular expression=",") -> (before substring=w4097:string, after substring=w4096:string)  [unwired: 1 in, 2 out]
                  "bs" <- w4097
                  "as" <- w4096
                  n3056 = Concatenate Strings(w4097, w4096) -> (w4093:string)
                  n3057 = property on="Temperature before test 2" class="DigNum (strict)"("Caption.Text"=w4093) -> ()  [unwired: 2 in, 2 out]
                  n3058 = property on="Temperature before test" class="DigNum (strict)"("Caption.Text"=w4093) -> ()  [unwired: 2 in, 2 out]
                  n3059 = Concatenate Strings(w4093, "=" ("string")) -> (→"String 34":string)
                }
                frame 40 {
                  n3060 = Match Pattern(string=w4105, regular expression=",") -> (before substring=w4104:string, after substring=w4103:string)  [unwired: 1 in, 2 out]
                  "bs" <- w4104
                  "as" <- w4103
                  n3061 = Concatenate Strings(w4104, w4103) -> (w4100:string)
                  n3062 = property on="Temperature after test 2" class="DigNum (strict)"("Caption.Text"=w4100) -> ()  [unwired: 2 in, 2 out]
                  n3063 = Concatenate Strings(w4100, "=" ("string")) -> (→"String 35":string)
                  n3064 = property on="Temperature after test" class="DigNum (strict)"("Caption.Text"=w4100) -> ()  [unwired: 2 in, 2 out]
                }
                frame 41 {
                  n3065 = property on="AVP" class="DigNum (strict)"("Caption.Text"=w4109) -> ()  [unwired: 2 in, 2 out]
                  n3066 = property on="AVP 2" class="DigNum (strict)"("Caption.Text"=w4109) -> ()  [unwired: 2 in, 2 out]
                  n3067 = Concatenate Strings(w4109, "=" ("string")) -> (→"String 36":string)
                }
                frame 42 {
                  n3068 = property on="MWSD" class="DigNum (strict)"("Caption.Text"=w4112) -> ()  [unwired: 2 in, 2 out]
                  n3069 = property on="MWSD 2" class="DigNum (strict)"("Caption.Text"=w4112) -> ()  [unwired: 2 in, 2 out]
                  n3070 = Concatenate Strings(w4112, "=" ("string")) -> (→"String 37":string)
                }
                frame 43 {
                  n3071 = property on="HCF 2" class="DigNum (strict)"("Caption.Text"=w4115) -> ()  [unwired: 2 in, 2 out]
                  n3072 = property on="HCF" class="DigNum (strict)"("Caption.Text"=w4115) -> ()  [unwired: 2 in, 2 out]
                  n3073 = Concatenate Strings(w4115, "=" ("string")) -> (→"String 38":string)
                }
                frame 44 {
                  n3074 = Concatenate Strings(w4117, "=" ("string")) -> (→"String 39":string)
                  n3075 = property on="WS1.4 2" class="DigNum (strict)"("Caption.Text"=w4117) -> ()  [unwired: 2 in, 2 out]
                  n3076 = property on="WS1.4" class="DigNum (strict)"("Caption.Text"=w4117) -> ()  [unwired: 2 in, 2 out]
                }
                frame 45 {
                  n3077 = property on="Save Results" class="Bool (strict)"("Boolean Text.Text"=w4119) -> ()  [unwired: 2 in, 2 out]
                }
                frame 46 {
                  n3078 = local write "S 47"(w4120) -> ()
                }
                frame 47 {
                  n3079 = local write "S 48"(w4121) -> ()
                }
                frame 48 {
                  n3080 = local write "S 49"(w4122) -> ()
                }
                frame 49 {
                  n3081 = local write "S 50"(w4123) -> ()
                }
                frame 50 {
                  n3082 = local write "S 51"(w4124) -> ()
                }
                frame 51 {
                  n3083 = local write "S 52"(w4125) -> ()
                }
                frame 52 {
                  n3084 = local write "S 53"(w4126) -> ()
                }
                frame 53 {
                  n3085 = local write "S 54"(w4127) -> ()
                }
                frame 54 {
                  n3086 = local write "S 55"(w4128) -> ()
                }
                frame 55 {
                  n3087 = local write "S 56"(w4129) -> ()
                }
                frame 56 {
                  n3088 = local write "S 57"(w4130) -> ()
                }
                frame 57 {
                  n3089 = local write "S 58"(w4131) -> ()
                }
                frame 58 {
                  n3090 = local write "S 59"(w4132) -> ()
                }
                frame 59 {
                  n3091 = local write "S 60"(w4133) -> ()
                }
                frame 60 {
                  n3092 = local write "S 62"(w4134) -> ()
                }
                frame 61 {
                  n3093 = local write "S 63"(w4135) -> ()
                }
                frame 62 {
                  n3094 = local write "S 64"(w4136) -> ()
                }
                frame 63 {
                  n3095 = local write "S 65"(w4137) -> ()
                }
                frame 64 {
                  n3096 = local write "S 66"(w4138) -> ()
                }
                frame 65 {
                  n3097 = local write "S 67"(w4139) -> ()
                }
                frame 66 {
                  n3098 = local write "S 68"(w4140) -> ()
                }
                frame 67 {
                  n3099 = local write "S 69"(w4141) -> ()
                }
                frame 68 {
                  n3100 = local write "S 70"(w4142) -> ()
                }
                frame 69 {
                  n3101 = local write "S 71"(w4143) -> ()
                }
                frame 70 {
                  n3102 = local write "S 72"(w4144) -> ()
                }
                frame 71 {
                  n3103 = local write "S 73"(w4145) -> ()
                }
                frame 72 {
                  n3104 = local write "S 74"(w4146) -> ()
                }
                frame 73 {
                  n3105 = local write "S 75"(w4147) -> ()
                }
                frame 74 {
                  n3106 = local write "S 76"(w4148) -> ()
                }
                frame 75 {
                  n3107 = local write "S 77"(w4149) -> ()
                }
                frame 76 {
                  n3108 = local write "S 78"(w4150) -> ()
                }
                frame 77 {
                  n3109 = local write "S 79"(w4151) -> ()
                }
                frame 79 {
                  n3110 = property on="Sample Temperature ( °C )" class="XYGraph (strict)"("Y Scale.Name Label.Text"=w4152) -> ()  [unwired: 2 in, 2 out]
                }
                frame 80 {
                  n3111 = local write "S 81"(w4153) -> ()
                  n3112 = property on="Humidity ( %RH )" class="XYGraph (strict)"("Y Scale.Name Label.Text"=w4153) -> ()  [unwired: 2 in, 2 out]
                }
                frame 78 {
                  n3113 = property on="Air Temperature  ( °C )" class="XYGraph (strict)"("X Scale.Name Label.Text"=w4154) -> ()  [unwired: 2 in, 2 out]
                  n3114 = property on="Humidity ( %RH )" class="XYGraph (strict)"("X Scale.Name Label.Text"=w4154) -> ()  [unwired: 2 in, 2 out]
                  n3115 = property on="Sample Temperature ( °C )" class="XYGraph (strict)"("X Scale.Name Label.Text"=w4154) -> ()  [unwired: 2 in, 2 out]
                  n3116 = property on="Coefficient Of Friction" class="XYGraph (strict)"("X Scale.Name Label.Text"=w4154) -> ()  [unwired: 2 in, 2 out]
                }
                frame 81 {
                  n3117 = property on="Air Temperature  ( °C )" class="XYGraph (strict)"("Y Scale.Name Label.Text"=w4155) -> ()  [unwired: 2 in, 2 out]
                }
                frame 82 {
                  n3118 = local write "S 84"(w4156) -> ()
                }
                frame 83 {
                  n3119 = local write "S 85"(w4157) -> ()
                }
                frame 84 {
                  n3120 = local write "S 86"(w4158) -> ()
                }
                frame 85 {
                  n3121 = local write "S 87"(w4159) -> ()
                }
                frame 86 {
                  n3122 = local write "S 88"(w4160) -> ()
                }
                frame 87 {
                }
                frame 88 {
                  n3123 = local write "S 90"(w4162) -> ()
                }
                frame 89 {
                  n3124 = local write "S 91"(w4163) -> ()
                }
                frame 90 {
